vi "Allign FFT Frames.vi"(8 "error in (no error)":errorcluster, 10 "FFT Size":u64, 11 "Unalligned FFT Amplitudes":refnum<class "2D Array f32.lvclass">) -> (0 "error out":errorcluster, 2 "FFT Size / 2":u64, 3 "Unalligned FFT Amplitudes":refnum<class "2D Array f32.lvclass">)   [LabVIEW 2020, in "GPU FFT Calculator.lvlib" / "GPU FFT Calculator.lvclass"]
uses:
  GPU FFT Calculator.lvclass
  <vilib>/Natan Biesmans/G2CPU GPU and CPU HPC Toolkit/G2CPU Libraries/Arrays/2DArray/f32/2D Array f32.lvclass
  C:/Program Files/National Instruments/LabVIEW 2026/vi.lib/Natan Biesmans/G2CPU GPU and CPU HPC Toolkit/G2CPU Libraries/Arrays/Array/Array Prototype.lvclass
  <vilib>/Natan Biesmans/G2CPU GPU and CPU HPC Toolkit/G2CPU Libraries/Arrays/Array/Array Prototype.lvclass/Array Prototype.ctl
  0b319cb6-abaa-46a7-a06c-11302e46d173.vi
  6bee67f9-5e91-4011-be87-fe97e14db18c.vi
  f5b4ccb4-8798-495e-bc62-027eeb16b7a2.vi
  65d9dd54-b85e-4bbc-b2bb-4cb06f857555.vi
  e6868991-1fd3-4bd5-88ae-a9f2f091ac6a.vi
  0b319cb6-abaa-46a7-a06c-11302e46d173.vi/ab6cfe59-c8ad-4da3-839b-8d02ec9e015f.vi
  <vilib>/Natan Biesmans/G2CPU GPU and CPU HPC Toolkit/G2CPU Libraries/Arrays/Array/G2CPU Get Array Pointer.vi
  6bee67f9-5e91-4011-be87-fe97e14db18c.vi/2e03f477-51b7-4ba0-bb4f-4f838f6557e6.vi
  6bee67f9-5e91-4011-be87-fe97e14db18c.vi/125d45d4-836b-469d-8a4a-6adb452f866d.vi
  6bee67f9-5e91-4011-be87-fe97e14db18c.vi/8038e9ed-2e71-4568-91ba-0d873494c5ed.vi
  f5b4ccb4-8798-495e-bc62-027eeb16b7a2.vi/5793b77b-c002-4ebf-9075-685617c95341.vi
  f5b4ccb4-8798-495e-bc62-027eeb16b7a2.vi/2ed3ef86-c00d-4d71-b84c-20267a6dfcf9.vi
  65d9dd54-b85e-4bbc-b2bb-4cb06f857555.vi/2e03f477-51b7-4ba0-bb4f-4f838f6557e6.vi
  65d9dd54-b85e-4bbc-b2bb-4cb06f857555.vi/125d45d4-836b-469d-8a4a-6adb452f866d.vi
  65d9dd54-b85e-4bbc-b2bb-4cb06f857555.vi/8038e9ed-2e71-4568-91ba-0d873494c5ed.vi
  e6868991-1fd3-4bd5-88ae-a9f2f091ac6a.vi/51c1d4c7-dece-4c02-9cce-b98611dadc4a.vi
  e6868991-1fd3-4bd5-88ae-a9f2f091ac6a.vi/3d9751b5-328d-444c-aff4-1d084998b389.vi
  0b319cb6-abaa-46a7-a06c-11302e46d173.vi/ab6cfe59-c8ad-4da3-839b-8d02ec9e015f.vi/313ec8c5-c203-475c-9de0-0583f6fb8b4d.vi
  6bee67f9-5e91-4011-be87-fe97e14db18c.vi/2e03f477-51b7-4ba0-bb4f-4f838f6557e6.vi/d8e2d9cc-c923-495e-b121-b6b84788c73f.vi
  6bee67f9-5e91-4011-be87-fe97e14db18c.vi/2e03f477-51b7-4ba0-bb4f-4f838f6557e6.vi/345e91f0-9a5e-4de4-af9c-133346717e4a.vi
  f5b4ccb4-8798-495e-bc62-027eeb16b7a2.vi/5793b77b-c002-4ebf-9075-685617c95341.vi/3e802c67-fb96-46a3-ae13-4994a8508b4f.vi
  f5b4ccb4-8798-495e-bc62-027eeb16b7a2.vi/5793b77b-c002-4ebf-9075-685617c95341.vi/5a50fc67-79e7-4972-80c2-92243cd53dd4.vi
  f5b4ccb4-8798-495e-bc62-027eeb16b7a2.vi/5793b77b-c002-4ebf-9075-685617c95341.vi/4b7910ad-0c4a-46e4-b1b3-c9721aeaa91e.vi
  f5b4ccb4-8798-495e-bc62-027eeb16b7a2.vi/2ed3ef86-c00d-4d71-b84c-20267a6dfcf9.vi/730f6c57-5c0b-4ee9-b61e-75067b25222b.vi
  f5b4ccb4-8798-495e-bc62-027eeb16b7a2.vi/2ed3ef86-c00d-4d71-b84c-20267a6dfcf9.vi/096b8799-7810-404e-baca-ba9279cec4bd.vi
  f5b4ccb4-8798-495e-bc62-027eeb16b7a2.vi/2ed3ef86-c00d-4d71-b84c-20267a6dfcf9.vi/0f1a5a47-bcc5-4796-ac31-8dfcfbc0d7d1.vi
  f5b4ccb4-8798-495e-bc62-027eeb16b7a2.vi/2ed3ef86-c00d-4d71-b84c-20267a6dfcf9.vi/89f12e17-3330-4b72-ad8f-8dd636660732.vi
  65d9dd54-b85e-4bbc-b2bb-4cb06f857555.vi/2e03f477-51b7-4ba0-bb4f-4f838f6557e6.vi/d8e2d9cc-c923-495e-b121-b6b84788c73f.vi
  65d9dd54-b85e-4bbc-b2bb-4cb06f857555.vi/2e03f477-51b7-4ba0-bb4f-4f838f6557e6.vi/345e91f0-9a5e-4de4-af9c-133346717e4a.vi
  <vilib>/Natan Biesmans/G2CPU GPU and CPU HPC Toolkit/ArrayFire Driver/VIs/Run as Multi Device.vi
  f5b4ccb4-8798-495e-bc62-027eeb16b7a2.vi/5793b77b-c002-4ebf-9075-685617c95341.vi/5a50fc67-79e7-4972-80c2-92243cd53dd4.vi/1b7cf390-2ae0-48f3-9bce-03c57eed6ee8.vi
  <vilib>/Natan Biesmans/G2CPU GPU and CPU HPC Toolkit/G2CPU Libraries/Arrays/1DArray/u32/1D Array u32.lvclass
  <vilib>/Natan Biesmans/G2CPU GPU and CPU HPC Toolkit/G2CPU Libraries/Arrays/1DArray/s32/1D Array s32.lvclass
  <vilib>/Natan Biesmans/G2CPU GPU and CPU HPC Toolkit/ArrayFire Driver/VIs/range.vi
  <vilib>/Natan Biesmans/G2CPU GPU and CPU HPC Toolkit/G2CPU Libraries/Arrays/Array/G2CPU Set Array Pointer.vi
  <vilib>/Natan Biesmans/G2CPU GPU and CPU HPC Toolkit/ArrayFire Driver/VIs/cast.vi
  <vilib>/Natan Biesmans/G2CPU GPU and CPU HPC Toolkit/ArrayFire Driver/VIs/lookup.vi
  <vilib>/Natan Biesmans/G2CPU GPU and CPU HPC Toolkit/ArrayFire Driver/subvi/Error Converter (ErrCode or Status).vi
  <vilib>/Natan Biesmans/G2CPU GPU and CPU HPC Toolkit/G2CPU Libraries/Arrays/SubVI/is 1D.vi
  <vilib>/Natan Biesmans/G2CPU GPU and CPU HPC Toolkit/ArrayFire Driver/VIs/add.vi
  <vilib>/Natan Biesmans/G2CPU GPU and CPU HPC Toolkit/ArrayFire Driver/VIs/join.vi
  <vilib>/Natan Biesmans/G2CPU GPU and CPU HPC Toolkit/G2CPU Libraries/Arrays/Array/Array Prototype.lvclass
  <vilib>/Natan Biesmans/G2CPU GPU and CPU HPC Toolkit/G2CPU Libraries/Arrays/DataTypes/I32/s32.lvclass
  <vilib>/Natan Biesmans/G2CPU GPU and CPU HPC Toolkit/G2CPU Libraries/Arrays/1DArray/1D Array Prototype.lvclass
  <vilib>/Natan Biesmans/G2CPU GPU and CPU HPC Toolkit/G2CPU Libraries/Arrays/DataTypes/U32/U32.lvclass
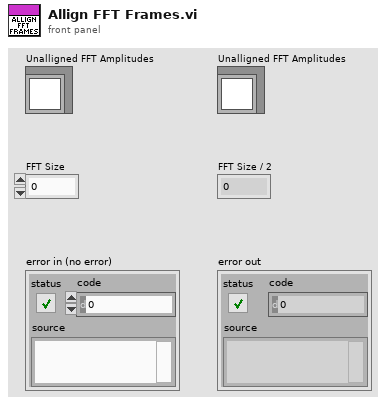
[diagram p1: front panel]
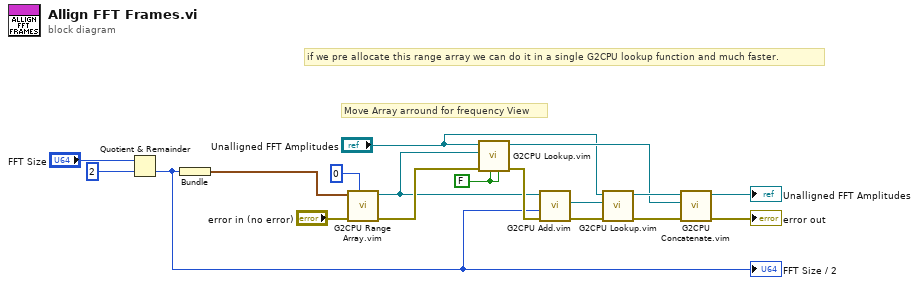
[diagram p0: block diagram]
diagram:
  w9 = FALSE ("Auto Release Array In (Enabled)")
  # "if we pre allocate this range array we can do it in a single G2CPU lookup function and much faster."
  # "Move Array arround for frequency View"
  n1 = Quotient & Remainder(x="FFT Size", y=u64 2 ("Datatype")) -> (floor(x/y)=w4:u64)  [unwired: 1 out]
  "FFT Size / 2" <- w4
  n2 = Bundle(w4) -> (w5:cluster{u64})  [unwired: 1 in]
  n3 = call "G2CPU Range Array.vim"("Datatype"=u32 0, "Error in"="error in (no error)", "Size"=w5) -> ("error out"=w13:errorcluster, "Array out"=w10:refnum<class "1D Array u32.lvclass">)  [unwired: 7 in]
  n4 = call "G2CPU Lookup.vim"("Auto Release Indices (Enabled)"=w9, "Auto Release Array In (Enabled)"=w9, "error in (no error)"=w13, "Indices (1D)"=w10, "Array In"="Unalligned FFT Amplitudes") -> ("error out"=w16:errorcluster, "Indexed Array"=w14:refnum<class "2D Array f32.lvclass">)  [unwired: 5 in]
  n5 = call "G2CPU Add.vim"("error in (no error)"=w16, "Array rhs"=w4, "Array lhs"=w10) -> ("error out"=w12:errorcluster, "Array Result"=w11:refnum<class "1D Array u32.lvclass">)  [unwired: 7 in]
  n6 = call "G2CPU Lookup.vim"("error in (no error)"=w12, "Indices (1D)"=w11, "Array In"="Unalligned FFT Amplitudes") -> ("error out"=w17:errorcluster, "Indexed Array"=w15:refnum<class "2D Array f32.lvclass">)  [unwired: 7 in]
  n7 = call "G2CPU Concatenate.vim"("error in (no error)"=w17, "Second Array In"=w14, "First Array In"=w15) -> ("error out"=→"error out":errorcluster, "Array out"=→"Unalligned FFT Amplitudes":refnum<class "2D Array f32.lvclass">)  [unwired: 7 in]
